vi "Get DeviceIDs.vi"(0 "DeviceID Array":T1[](array[typedef])) -> (1 "ES DeviceID":T1, 2 "PV DeviceID":T1, 3 "Gen DeviceID":T1)   [LabVIEW 2018, in "Alabama Power Remote Actor.lvlib" / "Alabama Power Remote.lvclass"]
uses:
  Alabama Power Remote.lvclass
  <vilib>/ORNL/CSEISMIC DDS/CSEISMIC DDS Base/Data Types/Controls/DeviceID.ctl
  <vilib>/ORNL/CSEISMIC DDS/CSEISMIC DDS Base/CSEISMIC DDS.lvclass
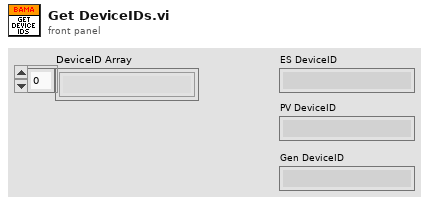
[diagram p1: front panel]
types:
  T1 = typedef "CSEISMIC DDS.lvlib/CSEISMIC DDS.lvclass/DeviceID.ctl" = string
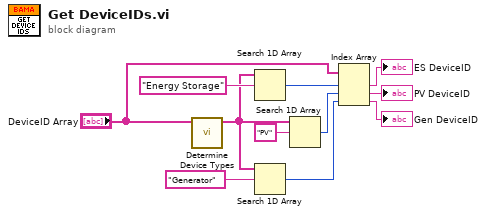
[diagram p0: block diagram]
diagram:
  n1 = call "Determine Device Types.vi"("DeviceIDs"="DeviceID Array") -> ("Device Classes"=w3:string[])  [unwired: 9 in]
  n2 = Search 1D Array(1D array=w3, element="Energy Storage") -> (index of element=w9:i32)  [unwired: 1 in]
  n3 = Search 1D Array(1D array=w3, element="Generator") -> (index of element=w2:i32)  [unwired: 1 in]
  n4 = Search 1D Array(1D array=w3, element="PV") -> (index of element=w6:i32)  [unwired: 1 in]
  n5 = Index Array(array="DeviceID Array", index #1=w9, index #2=w6, index #3=w2) -> (element #1=→"ES DeviceID":T1, element #2=→"PV DeviceID":T1, element #3=→"Gen DeviceID":T1)
